vi "迭代求最佳系数.vi"(8 "进位位":i32, 9 "标准值":dbl[](array[numeric])=[3686.0, 10980.0, 51980.0, 50600.0, 51200.0, 50500.0, 51200.0], 10 "1~4道":dbl[][](array[numeric])=[[673.0, 301.0, 1609.0, 2841.0], [1647.0, 849.0, 4700.0, 8552.0], [4816.0, 3132.0, 19355.0, 38642.0], [212735.0, 13241.0, 5087.0, 63.0], [217594.0, 44638.0, 40959.0, 249.0], [199449.0, 57659.0, 78920.0, 1630.0], [140863.0, 55251.0, 120310.0, 7683.0]], 11 "初始参数（布尔值都要为F，不要）":cluster{"参数":dbl, "须变动？":bool}[](array[cluster])=[{"参数"=0.4, "须变动？"=FALSE}, {"参数"=0.0, "须变动？"=FALSE}, {"参数"=0.12, "须变动？"=FALSE}, {"参数"=1.1, "须变动？"=FALSE}, {"参数"=800000.0, "须变动？"=FALSE}] {"参数" format="%#_13g"}) -> ()   [LabVIEW 2017]
uses:
  <vilib>/Analysis/NI_AALBase.lvlib
panel:
  in  "迭代次数(没用的)":i32=1
  out "最优参数":dbl[](array[numeric])
  out "最优索引":i32
  out "布尔数组":bool[](array[boolean])
  out "数组":bool[](array[boolean])
  in  "T+,F-":bool=TRUE
  out "计算值/标准值":dbl[](array[numeric])
  out "计算值":dbl[](array[numeric])=[673.0, 301.0, 1609.0, 2841.0]
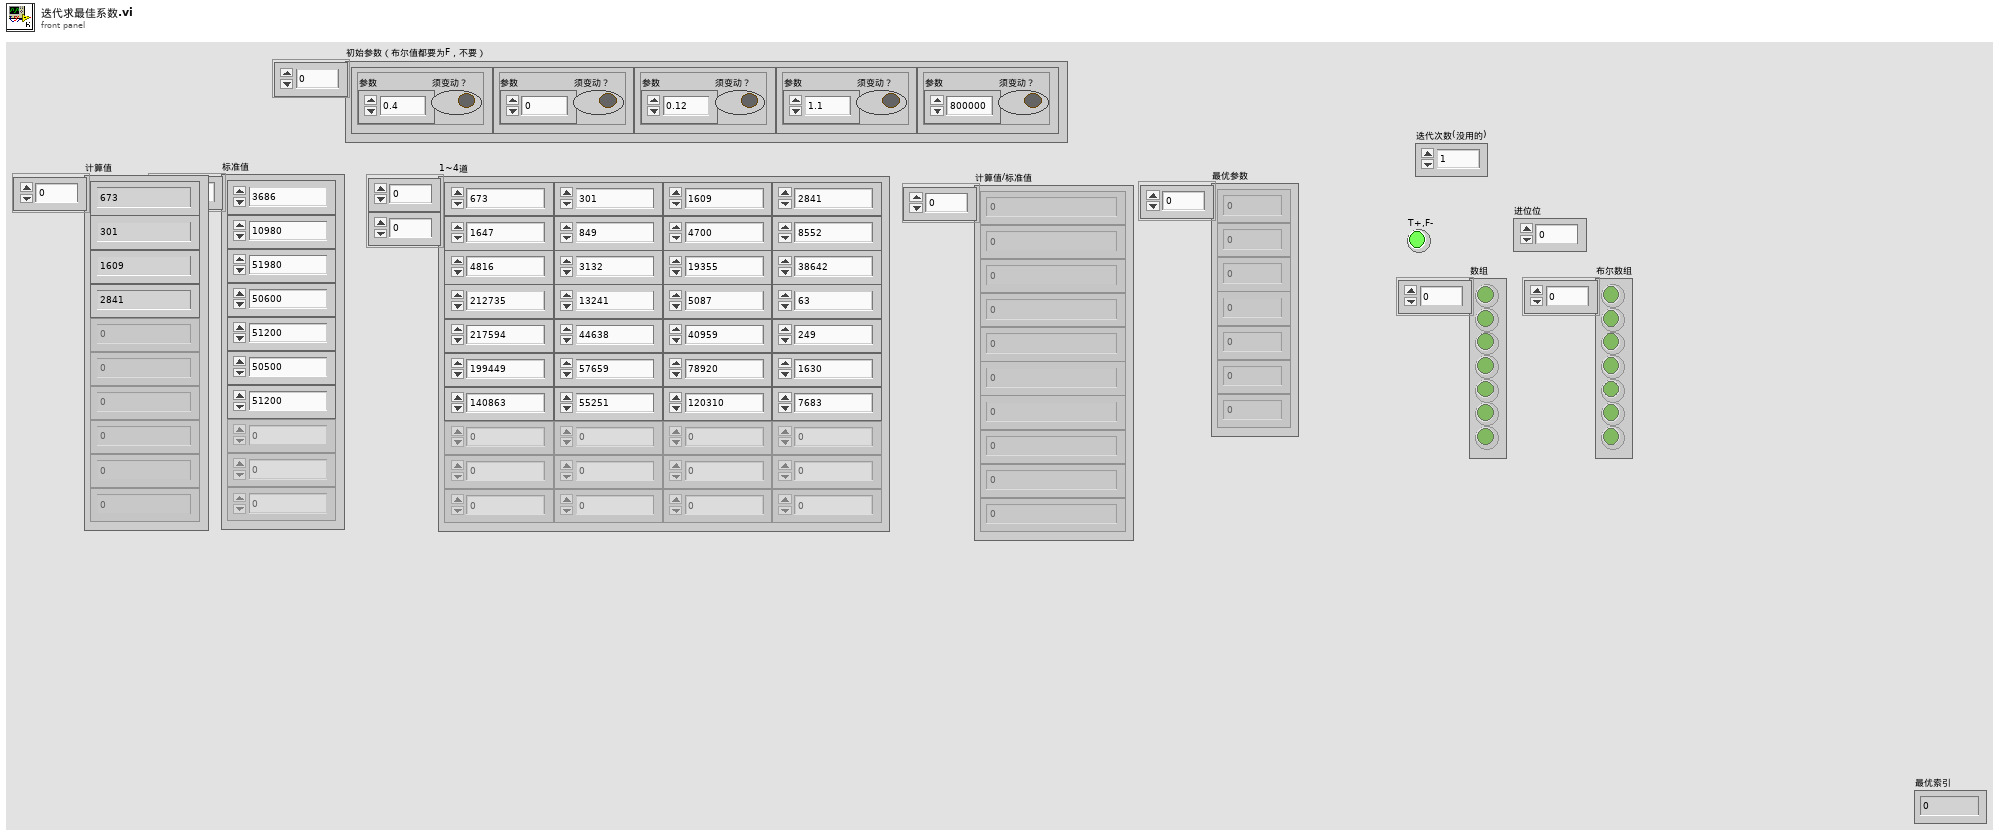
[diagram p1: front panel]
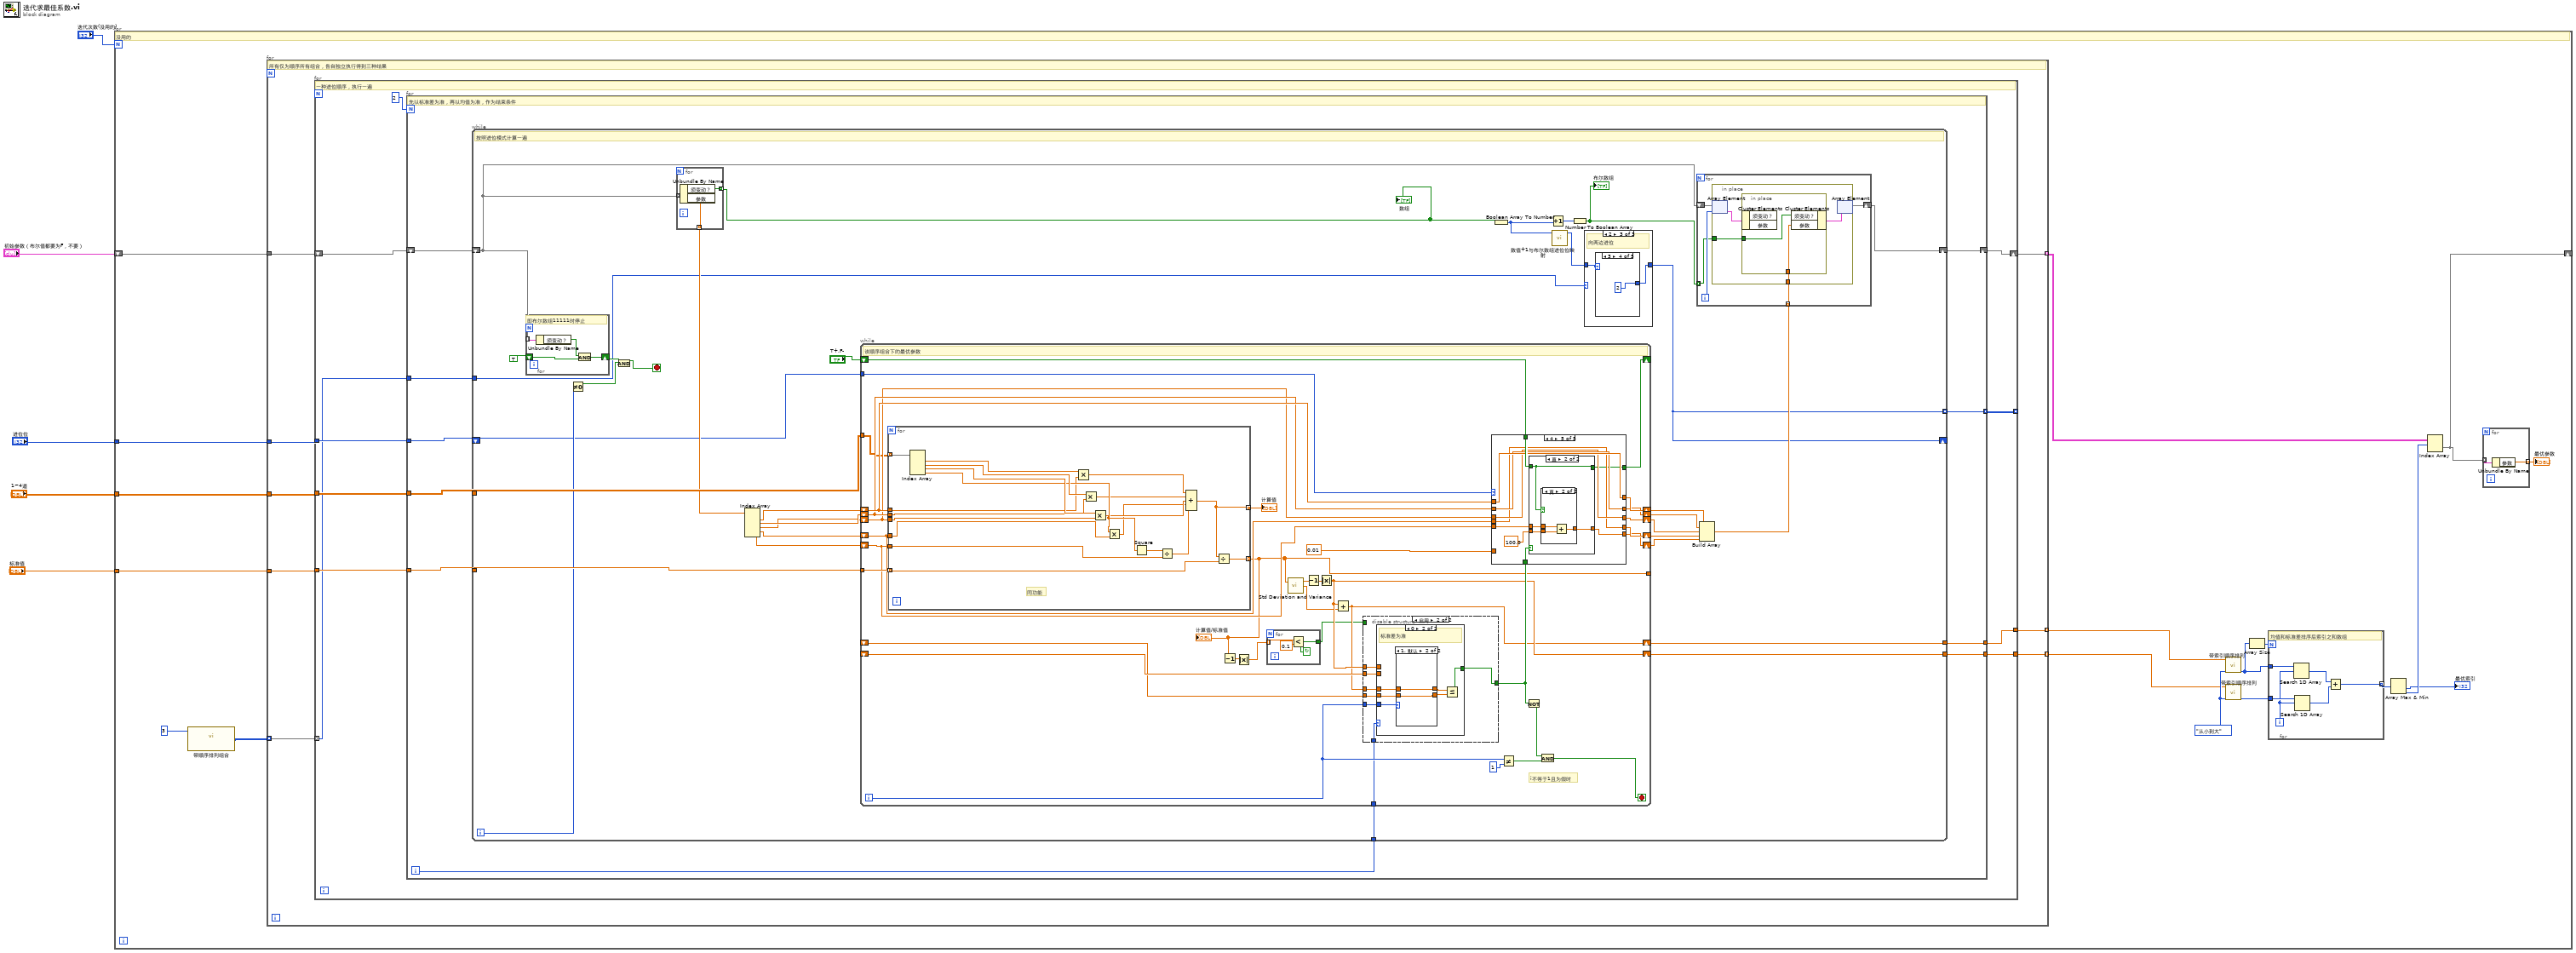
[diagram p0: block diagram]
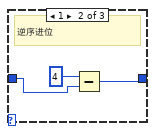
[diagram p3: hidden frame]
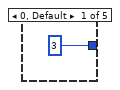
[diagram p4: hidden frame]
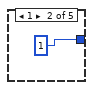
[diagram p5: hidden frame]
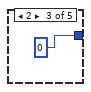
[diagram p6: hidden frame]
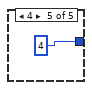
[diagram p7: hidden frame]
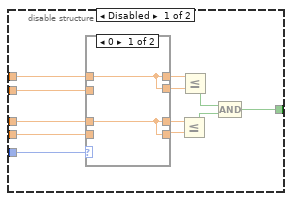
[diagram p8: hidden frame]
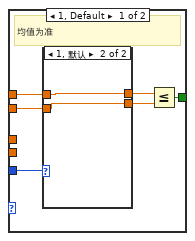
[diagram p10: hidden frame]
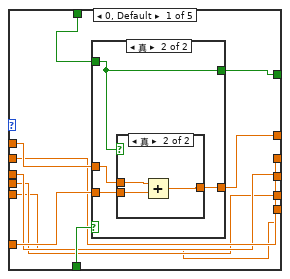
[diagram p13: hidden frame]
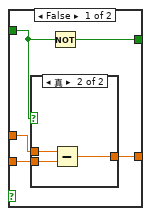
[diagram p14: hidden frame]
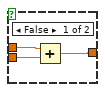
[diagram p15: hidden frame]
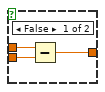
[diagram p16: hidden frame]
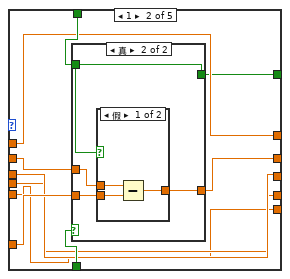
[diagram p17: hidden frame]
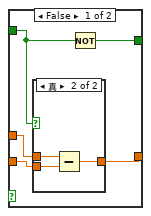
[diagram p18: hidden frame]
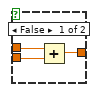
[diagram p19: hidden frame]
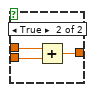
[diagram p20: hidden frame]
diagram:
  n1 = for {
    N: "迭代次数(没用的)" -> [_]
    tunnel: "1~4道" -> [w23]
    tunnel: "标准值" -> [w22]
    tunnel: "进位位" -> [w21]
    shift-right: [w9] -> _
    shift-left: "初始参数（布尔值都要为F，不要）" -> [w20]
    w19 = enum16{"从小到大", "从大到小"}."从小到大" ("排序模式")
    # "没用的"
    n2 = call "带顺序排列组合.vi"("数量"=3) -> ("组合o"=w6:i32[][])  [unwired: 10 in]
    n3 = for {
      tunnel: w23 -> [w39]
      tunnel: w22 -> [w38]
      tunnel: w21 -> [w37]
      tunnel: [w36] -> w11 mode=indexing
      tunnel: w20 -> [w35]
      tunnel: w6 -> [w34] mode=indexing
      tunnel: [w33] -> w13 mode=indexing
      tunnel: [w32] -> w12 mode=indexing
      # "所有仅为顺序所有组合，各自独立执行得到三种结果"
      n4 = for {
        tunnel: w39 -> [w49]
        tunnel: w38 -> [w48]
        tunnel: w37 -> [w47]
        tunnel: [w46] -> w33
        tunnel: [w45] -> w32
        shift-right: [w44] -> w36
        shift-left: w35 -> [w43]
        tunnel: [w41] -> _ mode=indexing
        tunnel: w34 -> [w40] mode=indexing
        # "一种进位顺序，执行一遍"
        n5 = for {
          N: 2 -> [_]
          tunnel: w49 -> [w58]
          tunnel: w48 -> [w57]
          tunnel: w47 -> [w56]
          tunnel: [w55] -> w46
          tunnel: [w54] -> w45
          shift-right: [w52] -> w44
          shift-left: w43 -> [w59]
          tunnel: w40 -> [w51]
          tunnel: [w50] -> w41 mode=indexing
          i -> [w53]
          # "先以标准差为准，再以均值为准，作为结束条件"
          n6 = while {
            shift-right: [w63] -> _
            shift-left: w56 -> [w60]
            tunnel: w58 -> [w92]
            tunnel: w57 -> [w91]
            shift-right: [w73] -> w52
            shift-left: w59 -> [w68]
            tunnel: [w63] -> w50 mode=indexing
            tunnel: [w67] -> w54
            tunnel: [w66] -> w55
            tunnel: w53 -> [w65]
            tunnel: w51 -> [w61]
            i -> [w62]
            stop <- w69 stop-if-true
            # "按照进位模式计算一遍"
            n7 = for {
              tunnel: w68 -> [w376] mode=indexing
              shift-right: [w373] -> w71
              shift-left: TRUE -> [w374]
              # "即布尔数组11111时停止"
              n8 = Unbundle By Name(w376) -> ("须变动？"=w375:bool)
              n9 = And(x=w375, y=w374) -> (x .and. y?=w373:bool)
            }
            n10 = Not Equal To 0?(x=w62) -> (x != 0?=w70:bool)
            n11 = And(x=w71, y=w70) -> (x .and. y?=w69:bool)
            n12 = for {
              tunnel: w68 -> [w371] mode=indexing
              tunnel: [w372] -> w90 mode=indexing
              tunnel: [w370] -> w76 mode=indexing
              n13 = Unbundle By Name(w371) -> ("须变动？"=w370:bool, "参数"=w372:dbl)
            }
            "数组" <- w76
            n14 = Index Array(array=w90) -> (element #1=w89:dbl, element #2=w88:dbl, element #3=w87:dbl, element #4=w86:dbl, element #5=w85:dbl)  [unwired: 5 in]
            n15 = while {
              tunnel: w92 -> [w124]
              tunnel: w91 -> [w149]
              shift-right: [w123] -> w67
              shift-left: _ -> [w144]
              shift-right: [w136] -> w83
              shift-left: w89 -> [w143]
              shift-right: [w135] -> w82
              shift-left: w88 -> [w142]
              shift-right: [w134] -> w81
              shift-left: w87 -> [w141]
              shift-right: [w133] -> w80
              shift-left: w86 -> [w140]
              shift-right: [w132] -> w79
              shift-left: w85 -> [w139]
              tunnel: w60 -> [w145]
              shift-right: [w125] -> _
              shift-left: "T+,F-" -> [w137]
              tunnel: [w118] -> _
              shift-right: [w120] -> w66
              shift-left: _ -> [w121]
              tunnel: w65 -> [w119]
              i -> [w131]
              stop <- w127 stop-if-true
              # "i不等于1且为假时"
              # "该顺序组合下的最优参数"
              n16 = for {
                tunnel: w124 -> [w369] mode=indexing
                tunnel: w149 -> [w364] mode=indexing
                tunnel: [w357] -> w118 mode=indexing
                tunnel: [w356] -> w148 mode=indexing
                tunnel: w143 -> [w355]
                tunnel: w142 -> [w354]
                tunnel: w141 -> [w353]
                tunnel: w140 -> [w352]
                tunnel: w139 -> [w351]
                # "同功能"
                n17 = Index Array(array=w369) -> (element #1=w368:dbl, element #2=w367:dbl, element #3=w366:dbl, element #4=w365:dbl)  [unwired: 4 in]
                n18 = Multiply(x=w368, y=w355) -> (x*y=w362:dbl)
                n19 = Multiply(x=w367, y=w354) -> (x*y=w361:dbl)
                n20 = Multiply(x=w366, y=w353) -> (x*y=w360:dbl)
                n21 = Multiply(x=w365, y=w352) -> (x*y=w359:dbl)
                n22 = Square(x=w365) -> (x^2=w363:dbl)
                n23 = Divide(x=w363, y=w351) -> (x/y=w358:dbl)
                n24 = Compound Arithmetic op=ADD(w362, w361, w360, w359, w358) -> (w356:dbl)
                n25 = Divide(x=w356, y=w364) -> (x/y=w357:dbl)
              }
              "计算值/标准值" <- w118
              "计算值" <- w148
              n26 = Decrement(x=w118) -> (x-1=w117:dbl[])
              n27 = Absolute Value(x=w117) -> (abs(x)=w116:dbl[])
              n28 = for {
                tunnel: w116 -> [w152] mode=indexing
                tunnel: [w150] -> w115
                stop <- w150 continue-if-true
                n29 = Less?(x=w152, y=0.1) -> (x < y?=w150:bool)
              }
              n30 = call <vilib>:"Std Deviation and Variance.vi"("X"=w118) -> ("mean"=w147:dbl, "standard deviation"=w122:dbl)  [unwired: 1 in, 1 out]
              n31 = Decrement(x=w147) -> (x-1=w146:dbl)
              n32 = Absolute Value(x=w146) -> (abs(x)=w123:dbl)
              n33 = Add(x=w123, y=w122) -> (x+y=w120:dbl)
              n34 = disable-structure shown="启用" {
                disable-tunnel: w144 -> [w161 w175]
                disable-tunnel: w131 -> [w160 w177]
                disable-tunnel: [w159 w171] -> w126
                disable-tunnel: w123 -> [w158 w176]
                disable-tunnel: w121 -> [w157 w173]
                disable-tunnel: w120 -> [w156 w174]
                disable-tunnel: w119 -> [_ w172]
                disable-tunnel: w115 -> [_ _]
                frame Disabled {
                  n35 = case shown="0" w160 {
                    tunnel: [w166 w170] -> w163
                    tunnel: w158 -> [w166 w170]
                    tunnel: [w166 w169] -> w162
                    tunnel: w161 -> [_ w169]
                    tunnel: w157 -> [_ w167]
                    tunnel: w156 -> [w165 w168]
                    tunnel: [w165 w168] -> w155
                    tunnel: [w165 w167] -> w154
                    frame 0 {
                    }
                    frame 1, Default {
                    }
                  }
                  n36 = Less Or Equal?(x=w155, y=w154) -> (x <= y?=w153:bool)
                  n37 = Less Or Equal?(x=w163, y=w162) -> (x <= y?=w164:bool)
                  n38 = Compound Arithmetic op=AND(w164, w153) -> (w159:bool)
                }
                frame Enabled {
                  n39 = case shown="0" w172 {
                    tunnel: w177 -> [w183 w192]
                    tunnel: w176 -> [w182 _]
                    tunnel: w175 -> [w181 _]
                    tunnel: [w178 w187] -> w171
                    tunnel: w174 -> [_ w191]
                    tunnel: w173 -> [_ w190]
                    frame 1, Default {
                      # "均值为准"
                      n40 = case shown="1, 默认" w183 {
                        tunnel: w182 -> [w184 w186]
                        tunnel: w181 -> [_ w185]
                        tunnel: [w184 w186] -> w180
                        tunnel: [w184 w185] -> w179
                        frame 0 {
                        }
                        frame 1, Default {
                        }
                      }
                      n41 = Less Or Equal?(x=w180, y=w179) -> (x <= y?=w178:bool)
                    }
                    frame 0 {
                      # "标准差为准"
                      n42 = case shown="1, 默认" w192 {
                        tunnel: w191 -> [w193 w195]
                        tunnel: w190 -> [_ w194]
                        tunnel: [w193 w195] -> w189
                        tunnel: [w193 w194] -> w188
                        frame 0 {
                        }
                        frame 1, Default {
                        }
                      }
                      n43 = Less Or Equal?(x=w189, y=w188) -> (x <= y?=w187:bool)
                    }
                  }
                }
              }
              n44 = case shown="4" w145 {
                tunnel: w143 -> [w204 w231 w262 w294 w326]
                tunnel: w142 -> [w200 w235 w261 w293 w325]
                tunnel: w141 -> [w199 w230 w266 w292 w324]
                tunnel: w140 -> [w198 w229 w260 w297 w323]
                tunnel: w139 -> [w197 w228 w259 w290 w328]
                tunnel: 0.01 ("结果") -> [w203 w234 w265 w296 _]
                tunnel: w137 -> [w205 w236 w267 w298 w327]
                tunnel: w126 -> [w202 w233 w264 w295 w321]
                tunnel: [w201 w231 w262 w294 w326] -> w136
                tunnel: [w200 w232 w261 w293 w325] -> w135
                tunnel: [w199 w230 w263 w292 w324] -> w134
                tunnel: [w198 w229 w260 w291 w323] -> w133
                tunnel: [w197 w228 w259 w290 w322] -> w132
                tunnel: [w196 w227 w258 w289 w320] -> w125
                frame 0, Default {
                  n45 = case shown="真" w202 {
                    tunnel: w204 -> [w210 w219]
                    tunnel: w205 -> [w207 w217]
                    tunnel: w203 -> [w209 w220]
                    tunnel: [w208 w218] -> w201
                    tunnel: [w206 w217] -> w196
                    frame False {
                      n46 = case shown="真" w207 {
                        tunnel: w209 -> [w212 w216]
                        tunnel: w210 -> [w213 w215]
                        tunnel: [w211 w214] -> w208
                        frame False {
                          n47 = Add(x=w213, y=w212) -> (x+y=w211:dbl)
                        }
                        frame True {
                          n48 = Subtract(x=w215, y=w216) -> (x-y=w214:dbl)
                        }
                      }
                      n49 = Not(x=w207) -> (.not. x?=w206:bool)
                    }
                    frame True {
                      n50 = case shown="真" w217 {
                        tunnel: w220 -> [w223 w225]
                        tunnel: w219 -> [w222 w226]
                        tunnel: [w221 w224] -> w218
                        frame False {
                          n51 = Subtract(x=w222, y=w223) -> (x-y=w221:dbl)
                        }
                        frame True {
                          n52 = Add(x=w226, y=w225) -> (x+y=w224:dbl)
                        }
                      }
                    }
                  }
                }
                frame 1 {
                  n53 = case shown="真" w233 {
                    tunnel: w235 -> [w241 w250]
                    tunnel: w236 -> [w238 w248]
                    tunnel: w234 -> [w240 w251]
                    tunnel: [w239 w249] -> w232
                    tunnel: [w237 w248] -> w227
                    frame False {
                      n54 = case shown="真" w238 {
                        tunnel: w240 -> [w243 w247]
                        tunnel: w241 -> [w244 w246]
                        tunnel: [w242 w245] -> w239
                        frame False {
                          n55 = Add(x=w244, y=w243) -> (x+y=w242:dbl)
                        }
                        frame True {
                          n56 = Subtract(x=w246, y=w247) -> (x-y=w245:dbl)
                        }
                      }
                      n57 = Not(x=w238) -> (.not. x?=w237:bool)
                    }
                    frame True {
                      n58 = case shown="假" w248 {
                        tunnel: w251 -> [w254 w256]
                        tunnel: w250 -> [w253 w257]
                        tunnel: [w252 w255] -> w249
                        frame False {
                          n59 = Subtract(x=w253, y=w254) -> (x-y=w252:dbl)
                        }
                        frame True {
                          n60 = Add(x=w257, y=w256) -> (x+y=w255:dbl)
                        }
                      }
                    }
                  }
                }
                frame 2 {
                  n61 = case shown="真" w264 {
                    tunnel: w266 -> [w272 w281]
                    tunnel: w267 -> [w269 w279]
                    tunnel: w265 -> [w271 w282]
                    tunnel: [w270 w280] -> w263
                    tunnel: [w268 w279] -> w258
                    frame False {
                      n62 = case shown="真" w269 {
                        tunnel: w271 -> [w274 w278]
                        tunnel: w272 -> [w275 w277]
                        tunnel: [w273 w276] -> w270
                        frame False {
                          n63 = Add(x=w275, y=w274) -> (x+y=w273:dbl)
                        }
                        frame True {
                          n64 = Subtract(x=w277, y=w278) -> (x-y=w276:dbl)
                        }
                      }
                      n65 = Not(x=w269) -> (.not. x?=w268:bool)
                    }
                    frame True {
                      n66 = case shown="假" w279 {
                        tunnel: w282 -> [w285 w287]
                        tunnel: w281 -> [w284 w288]
                        tunnel: [w283 w286] -> w280
                        frame False {
                          n67 = Subtract(x=w284, y=w285) -> (x-y=w283:dbl)
                        }
                        frame True {
                          n68 = Add(x=w288, y=w287) -> (x+y=w286:dbl)
                        }
                      }
                    }
                  }
                }
                frame 3 {
                  n69 = case shown="真" w295 {
                    tunnel: w297 -> [w303 w312]
                    tunnel: w298 -> [w300 w310]
                    tunnel: w296 -> [w302 w313]
                    tunnel: [w301 w311] -> w291
                    tunnel: [w299 w310] -> w289
                    frame False {
                      n70 = case shown="真" w300 {
                        tunnel: w302 -> [w305 w309]
                        tunnel: w303 -> [w306 w308]
                        tunnel: [w304 w307] -> w301
                        frame False {
                          n71 = Add(x=w306, y=w305) -> (x+y=w304:dbl)
                        }
                        frame True {
                          n72 = Subtract(x=w308, y=w309) -> (x-y=w307:dbl)
                        }
                      }
                      n73 = Not(x=w300) -> (.not. x?=w299:bool)
                    }
                    frame True {
                      n74 = case shown="假" w310 {
                        tunnel: w313 -> [w316 w318]
                        tunnel: w312 -> [w315 w319]
                        tunnel: [w314 w317] -> w311
                        frame False {
                          n75 = Subtract(x=w315, y=w316) -> (x-y=w314:dbl)
                        }
                        frame True {
                          n76 = Add(x=w319, y=w318) -> (x+y=w317:dbl)
                        }
                      }
                    }
                  }
                }
                frame 4 {
                  n77 = case shown="真" w321 {
                    tunnel: w328 -> [w334 w343]
                    tunnel: w327 -> [w331 w341]
                    tunnel: 100.0 ("结果") -> [w333 w344]
                    tunnel: [w332 w342] -> w322
                    tunnel: [w330 w341] -> w320
                    frame False {
                      n78 = case shown="假" w331 {
                        tunnel: w333 -> [w336 w340]
                        tunnel: w334 -> [w337 w339]
                        tunnel: [w335 w338] -> w332
                        frame False {
                          n79 = Add(x=w337, y=w336) -> (x+y=w335:dbl)
                        }
                        frame True {
                          n80 = Subtract(x=w339, y=w340) -> (x-y=w338:dbl)
                        }
                      }
                      n81 = Not(x=w331) -> (.not. x?=w330:bool)
                    }
                    frame True {
                      n82 = case shown="真" w341 {
                        tunnel: w344 -> [w347 w349]
                        tunnel: w343 -> [w346 w350]
                        tunnel: [w345 w348] -> w342
                        frame False {
                          n83 = Subtract(x=w346, y=w347) -> (x-y=w345:dbl)
                        }
                        frame True {
                          n84 = Add(x=w350, y=w349) -> (x+y=w348:dbl)
                        }
                      }
                    }
                  }
                }
              }
              n85 = Not Equal?(x=w131, y=1) -> (x != y?=w129:bool)
              n86 = Not(x=w126) -> (.not. x?=w128:bool)
              n87 = And(x=w128, y=w129) -> (x .and. y?=w127:bool)
            }
            n88 = Boolean Array To Number(Boolean array=w76) -> (number=w75:u32)
            n89 = Increment(x=w75) -> (x+1=w78:u32)
            n90 = call "数值+1与布尔数组进位位映射.vi"("U8整型"=w75) -> ("进位位"=w64:i32)  [unwired: 10 in]
            n91 = Number To Boolean Array(number=w78) -> (Boolean array=w77:bool[])
            "布尔数组" <- w77
            n92 = case shown="2" w61 {
              tunnel: w64 -> [w93 w95 w98]
              tunnel: [w93 w94 w97] -> w63
              frame 0, Default {
                # "顺序进位"
              }
              frame 1 {
                # "逆序进位"
                n93 = Subtract(x=4, y=w95) -> (x-y=w94:i32)
              }
              frame 2 {
                # "向两边进位"
                n94 = case shown="3" w98 {
                  tunnel: [3 ("进位位") 1 ("进位位") 0 ("进位位") 2 ("进位位") 4 ("进位位")] -> w97
                  frame 0, Default {
                  }
                  frame 1 {
                  }
                  frame 2 {
                  }
                  frame 3 {
                  }
                  frame 4 {
                  }
                }
              }
            }
            n95 = Build Array(w83, w82, w81, w80, w79) -> (w74:dbl[])
            n96 = for {
              tunnel: w77 -> [w107] mode=indexing
              tunnel: w74 -> [w105] mode=indexing
              shift-right: [w106] -> w73
              shift-left: w68 -> [w104]
              i -> [w108]
              n97 = in-place {
                in-place-border: w107 -> [w111]
                in-place-border: w105 -> [w109]
                n98 = in-place-array #1(w104, w108) -> (w112:cluster{"参数":dbl, "须变动？":bool})
                n99 = in-place {
                  in-place-border: w111 -> [w114]
                  in-place-border: w109 -> [w113]
                  n100 = in-place-cluster #2(w112) -> ()  [unwired: 2 out]
                  n101 = in-place-cluster #2("须变动？"=w114, "参数"=w113) -> (w110:cluster{"参数":dbl, "须变动？":bool})
                }
                n102 = in-place-array #1(w110) -> (w106:cluster{"参数":dbl, "须变动？":bool}[])  [unwired: 1 out]
              }
            }
          }
        }
      }
    }
    n103 = call "带索引顺序排列.vi"("排序模式"=w19, "数组"=w13) -> ("索引映射"=w17:i32[])  [unwired: 8 in, 1 out]
    n104 = call "带索引顺序排列.vi"("排序模式"=w19, "数组"=w12) -> ("索引映射"=w14:i32[])  [unwired: 8 in, 1 out]
    n105 = Array Size(array=w17) -> (size(s)=w18:i32)
    n106 = for {
      N: w18 -> [_]
      tunnel: w17 -> [w31]
      tunnel: w14 -> [w30]
      tunnel: [w26] -> w15 mode=indexing
      i -> [w29]
      # "均值和标准差排序后索引之和数组"
      n107 = Search 1D Array(1D array=w31, element=w29) -> (index of element=w28:i32)  [unwired: 1 in]
      n108 = Search 1D Array(1D array=w30, element=w29) -> (index of element=w27:i32)  [unwired: 1 in]
      n109 = Add(x=w28, y=w27) -> (x+y=w26:i32)
    }
    n110 = Array Max & Min(array=w15) -> (min value=→"最优索引":i32, min index (indices)=w16:i32)  [unwired: 2 out]
    n111 = Index Array(array=w11, index (row)=w16) -> (element=w9:cluster{"参数":dbl, "须变动？":bool}[])  [unwired: 1 in]
    n112 = for {
      tunnel: w9 -> [w25] mode=indexing
      tunnel: [w24] -> w10 mode=indexing
      n113 = Unbundle By Name(w25) -> ("参数"=w24:dbl)
    }
    "最优参数" <- w10
  }
